vi "Read shared variable IR_data.vi"(8 "error in (no error)":errorcluster, 11 "VIS-NIR_STRESING_NEW in":refnum<class "VIS-NIR_STRESING_NEW.lvclass">) -> (0 "error out":errorcluster, 2 "shared variable IR_data":refnum<k21>, 3 "VIS-NIR_STRESING_NEW out":refnum<class "VIS-NIR_STRESING_NEW.lvclass">)   [LabVIEW 2020, in "VIS-NIR_STRESING_NEW.lvclass"]
uses:
  VIS-NIR_STRESING_NEW/VIS-NIR_STRESING_NEW.lvclass
  VIS-NIR_STRESING_NEW/VIS-NIR_STRESING_NEW.lvclass/VIS-NIR_STRESING_NEW.ctl
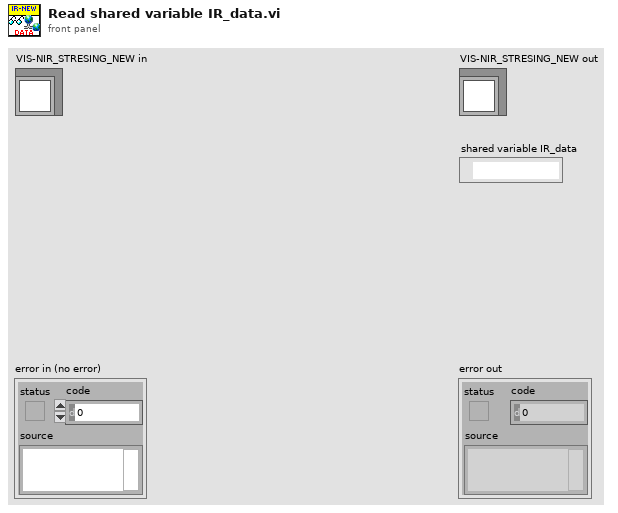
[diagram p1: front panel]
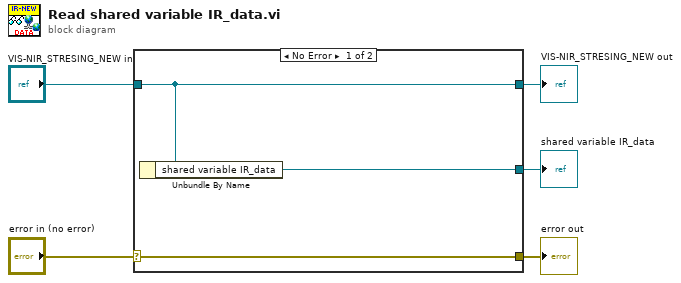
[diagram p0: block diagram]
diagram:
  n1 = case shown="No Error" "error in (no error)" {
    selector: "error in (no error)" -> [w8 w9]
    tunnel: [w8 w9] -> w4
    tunnel: [w7 w10] -> w2
    tunnel: "VIS-NIR_STRESING_NEW in" -> [w7 w10]
    tunnel: [w6 _] -> w1
    frame No Error {
      n2 = Unbundle By Name(w7) -> ("shared variable IR_data"=w6:refnum<k21>)
    }
    frame Error {
    }
  }
  "error out" <- w4
  "VIS-NIR_STRESING_NEW out" <- w2
  "shared variable IR_data" <- w1
